vi "VIremotePalette.vi"   [LabVIEW 2011]
uses:
  <vilib>/Palette API/Palette Menu/Public Type Define/Item.ctl
  <vilib>/Palette API/Palette Menu/Public Type Define/Palette type.ctl
  <vilib>/Palette API/Palette Menu/Palette Menu.lvlib
panel:
  # "Creating palettes..."
types:
  T1 = typedef "Palette Menu.lvlib/Item.ctl" = cluster{"item path":path, "library path (.lvlib)":path, "use default lvlib palette":bool, "short name":string, "place VI contents":bool, "hide synchronized item":bool, "reserve spot for synch item":bool, "configure when placing VI contents":bool}
  T2 = typedef "imagedata.ctl" = cluster{"image type":i32, "image depth":i32, "image":u8[], "mask":u8[], "colors":u32[], "Rectangle":cluster{"left":i16, "top":i16, "right":i16, "bottom":i16}}
  T3 = typedef "Palette Menu.lvlib/View Format.ctl" = u16
  T4 = typedef "Palette Menu.lvlib/Palette type.ctl" = i32
  T5 = cluster{"Menu name":string, "Strings [] VIs":string[], "View Format":T3, "Palette Type":T4}[]
  T6 = typedef "Palette Menu.lvlib/Palette Data.ctl" = cluster{"display name":string, "view format":T3, "palette width":i16, "items":T7, "256 color icon":picture, "B&W color icon":picture, "help information":T8, "palette description":string, "synchronize information":T9}
  T7 = typedef "Palette Menu.lvlib/Items.ctl" = T1[]
  T8 = typedef "Palette Menu.lvlib/Help Info.ctl" = cluster{"help tag":string, "help file path ":path}
  T9 = typedef "Palette Menu.lvlib/Synchronize Info.ctl" = cluster{"synchronize with directory":bool, "synchronize directory path":path}
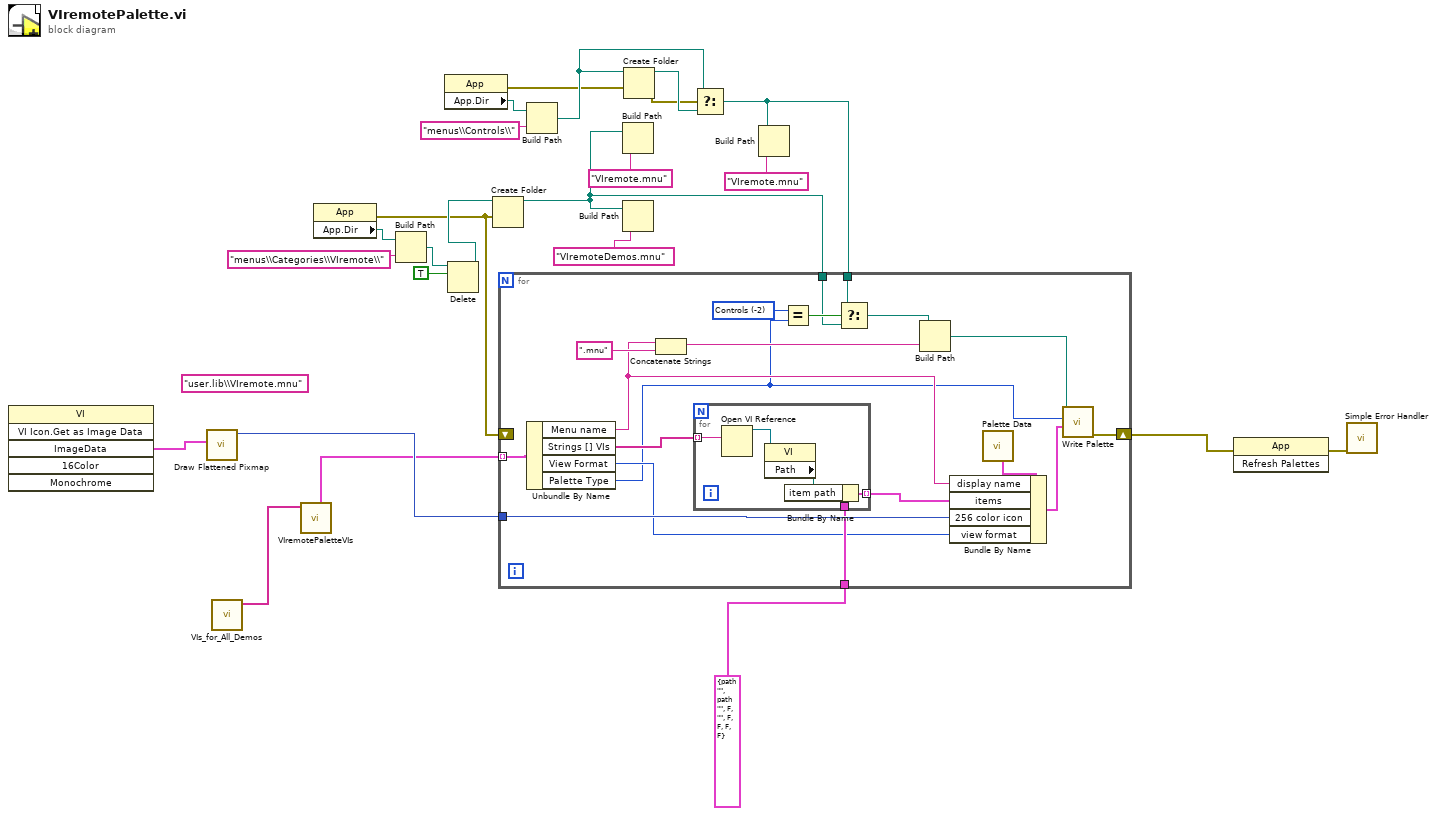
[diagram p0: block diagram]
diagram:
  (unwired) "user.lib\\VIremote.mnu" ("name or relative path")
  n1 = invoke class="VI" method="VI Icon.Get as Image Data"() -> ("ImageData"=w22:T2)  [unwired: 6 in, 5 out]
  n2 = call <vilib>:"Draw Flattened Pixmap.vi"("image data"=w22) -> ("new picture"=w13:picture)  [unwired: 1 in, 7 out]
  n3 = call "VIs_for_All_Demos.vi"() -> ("Strings []"=w7:string[])  [unwired: 1 in, 10 out]
  n4 = call "VIremotePaletteVIs.vi"("Strings [] Demo VIs"=w7) -> ("Array"=w6:T5)  [unwired: 10 out]
  n5 = property class="App"() -> (error out=w4:errorcluster, "App.Dir"=w24:path)  [unwired: 2 in, 1 out]
  n6 = Build Path(base path=w24, name or relative path="menus\\Categories\\VIremote\\") -> (appended path=w10:path)
  n7 = property class="App"() -> (error out=w16:errorcluster, "App.Dir"=w14:path)  [unwired: 2 in, 1 out]
  n8 = Delete(path (use dialog)=w10, entire hierarchy (F)=TRUE) -> (deleted path=w9:path)  [unwired: 1 in, 4 out]
  n9 = Create Folder(path (use dialog)=w9, error in=w4) -> (created path=w1:path)  [unwired: 3 out]
  n10 = Build Path(base path=w14, name or relative path="menus\\Controls\\") -> (appended path=w19:path)
  n11 = Build Path(base path=w1, name or relative path="VIremote.mnu") -> ()  [unwired: 1 out]
  n12 = Build Path(base path=w1, name or relative path="VIremoteDemos.mnu") -> ()  [unwired: 1 out]
  n13 = Create Folder(path (use dialog)=w19, error in=w16) -> (created path=w20:path, error out=w18:errorcluster)  [unwired: 2 out]
  n14 = Select(t=w19, s=w18, f=w20) -> (s? t:f=w2:path)
  n15 = for {
    tunnel: w13 -> [w41]
    tunnel: w6 -> [w40] mode=indexing
    tunnel: T1 {"item path"=path "", "library path (.lvlib)"=path "", "use default lvlib palette"=FALSE, "short name"="", "place VI contents"=FALSE, "hide synchronized item"=FALSE, "reserve spot for synch item"=FALSE, "configure when placing VI contents"=FALSE} ("Items") -> [w33]
    shift-right: [w32] -> w3
    shift-left: w4 -> [_]
    tunnel: w2 -> [w27]
    tunnel: w1 -> [w26]
    w29 = T4 -2 items=["Functions"=-1, "Controls"=-2] ("x")
    n16 = Unbundle By Name(w40) -> ("Menu name"=w37:string, "Strings [] VIs"=w39:string[], "View Format"=w31:T3, "Palette Type"=w30:T4)
    n17 = Concatenate Strings(w37, ".mnu" ("string")) -> (w36:string)
    n18 = for {
      tunnel: w39 -> [w48] mode=indexing
      tunnel: w33 -> [w45]
      tunnel: [w44] -> w34 mode=indexing
      n19 = Open VI Reference(vi path=w48) -> (vi reference=w47:refnum<vi>)  [unwired: 1 in, 5 out]
      n20 = property class="VI"(reference=w47) -> ("Path"=w46:path)  [unwired: 1 in, 2 out]
      n21 = Bundle By Name(cluster=w45, "item path"=w46) -> (w44:T1)
    }
    n22 = Equal?(x=w29, y=w30) -> (x = y?=w28:bool)
    n23 = Select(t=w27, s=w28, f=w26) -> (s? t:f=w25:path)
    n24 = Build Path(base path=w25, name or relative path=w36) -> (appended path=w35:path)
    n25 = call <vilib>:"Palette Data.vi"() -> ("Palette  Data"=w43:T6)  [unwired: 11 out]
    n26 = Bundle By Name(cluster=w43, "display name"=w37, "items"=w34, "256 color icon"=w41, "view format"=w31) -> (w42:T6)
    n27 = call <vilib>:"Write Palette.vi"("palette data"=w42, "palette type"=w30, "palette path"=w35) -> ("error out"=w32:errorcluster)  [unwired: 2 in, 6 out]
  }
  n28 = Build Path(base path=w2, name or relative path="VIremote.mnu") -> ()  [unwired: 1 out]
  n29 = invoke class="App" method="Refresh Palettes"(error in=w3) -> (error out=w23:errorcluster)  [unwired: 2 in, 2 out]
  n30 = call <vilib>:"Simple Error Handler.vi"("error in (no error)"=w23) -> ()  [unwired: 1 in, 8 out]
